vi "Get Library Item Path.vi"(8 "error in (no error)":errorcluster, 11 "Library":refnum<vi>) -> (0 "error out":errorcluster, 2 "Path":path, 3 "Library":refnum<vi>)   [LabVIEW 2019, in "gRPC Template Creation Utility.lvlib"]
uses:
  gRPC Template Creation Utility.lvlib
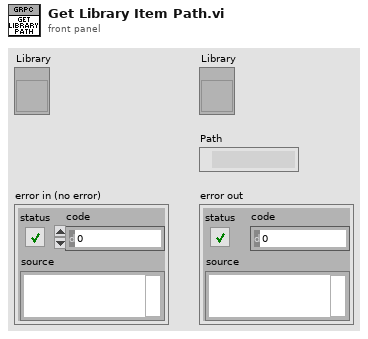
[diagram p1: front panel]
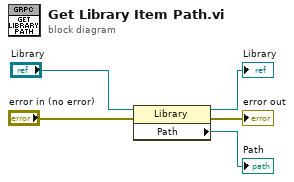
[diagram p0: block diagram]
diagram:
  n1 = property class="Library"(reference="Library", error in="error in (no error)") -> (reference out=→"Library":refnum<vi>, error out=→"error out":errorcluster, "Path"=→"Path":path)
